vi "Init GPIO.vi"(7 "GPIO #":T3=-1, 8 "error in (no error)":errorcluster, 9 "GPIO Pull (None)":T2, 10 "GPIO Direction":T1, 11 "Session in":refnum<class "Session.lvclass">) -> (0 "error out":errorcluster, 2 "GPIO":refnum<class "GPIO.lvclass">, 3 "Session out":refnum<class "Session.lvclass">)   [LabVIEW 2020, in "CTI.lvlib" / "Session.lvclass"]
uses:
  Session.lvclass
  GPIO Number.ctl
  GPIO/GPIO.lvclass
  GPIO Pull.ctl
  GPIO Direction.ctl
  CTI.lvlib
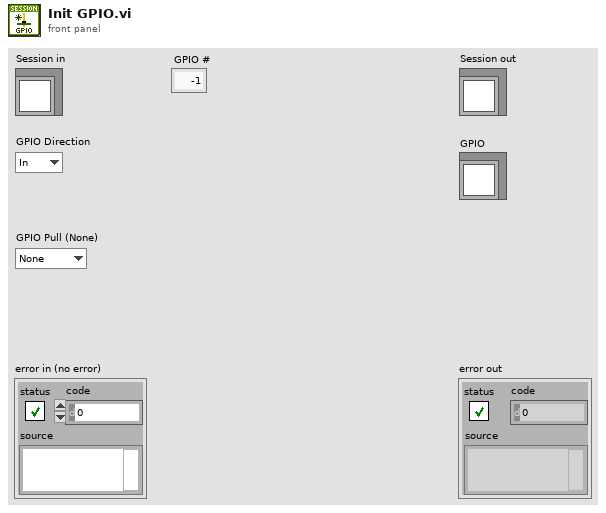
[diagram p1: front panel]
types:
  T1 = typedef "CTI.lvlib/GPIO Direction.ctl" = enum16{"In", "Out"}
  T2 = typedef "CTI.lvlib/GPIO Pull.ctl" = enum16{"None", "Up", "Down", "Both"}
  T3 = typedef "CTI.lvlib/GPIO Number.ctl" = i8
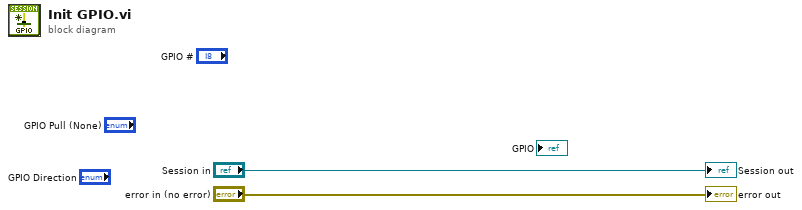
[diagram p0: block diagram]
diagram:
  "error out" <- "error in (no error)"
  "Session out" <- "Session in"
